vi "insert_doubles_array_example.vi"() -> ()   [LabVIEW 2020, in "Data.PG.lvclass"]
uses:
  Data.PG.lvclass
panel:
  in  "How many points":i32
  in  "Data.PG in":refnum<class "Data.PG.lvclass">
  out "Data.PG out":refnum<class "Data.PG.lvclass">
  in  "milliseconds to wait between points":u32
  in  "paths":string[](array[string])
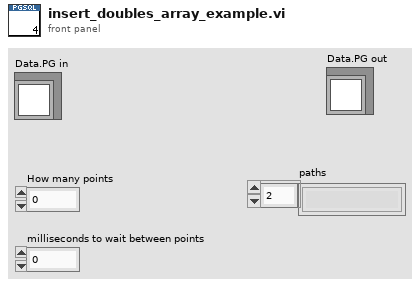
[diagram p1: front panel]
types:
  T1 = cluster{"host":string, "port":string, "user":string, "dbname":string, "password":string}
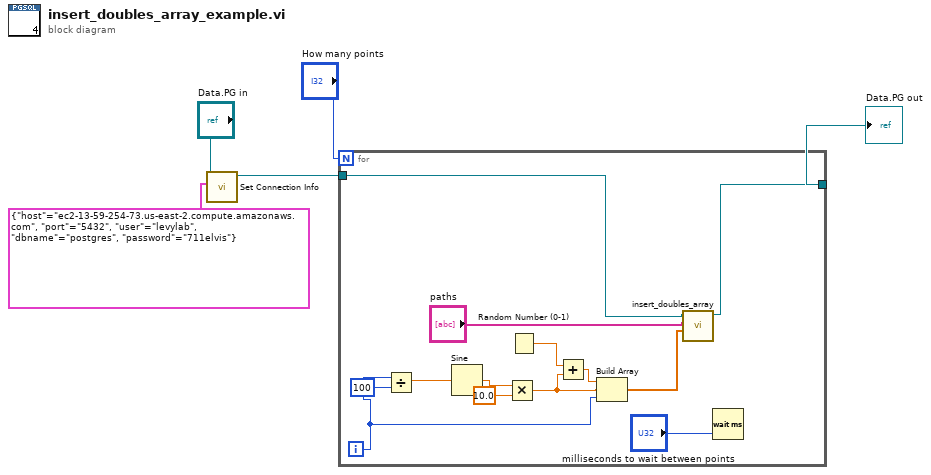
[diagram p0: block diagram]
diagram:
  n1 = call "Set Connection Info.vi"("connection info"=T1 {"host"="ec2-13-59-254-73.us-east-2.compute.amazonaws.com", "port"="5432", "user"="levylab", "dbname"="postgres", "password"="711elvis"}, "Data.PG in"="Data.PG in") -> ("Data.PG out"=w3:refnum<class "Data.PG.lvclass">)  [unwired: 8 in, 1 out]
  n2 = for {
    N: "How many points" -> [_]
    tunnel: w3 -> [w9]
    tunnel: [w6] -> w2
    i -> [w10]
    n3 = Divide(x=w10, y=100) -> (x/y=w18:dbl)
    n4 = Sine(x=w18) -> (sin(x)=w16:dbl)
    n5 = Multiply(x=w16, y=10.0) -> (x*y=w11:dbl)
    n6 = Random Number (0-1)() -> (number: 0 to 1=w14:dbl)
    n7 = Add(x=w14, y=w11) -> (x+y=w12:dbl)
    n8 = Build Array(w12, w11, w10) -> (w7:dbl[])
    n9 = call "insert_doubles_array.vi"("Values"=w7, "paths"="paths", "Data.PG in"=w9) -> ("Data.PG out"=w6:refnum<class "Data.PG.lvclass">)  [unwired: 7 in, 1 out]
    n10 = Wait (ms)(milliseconds to wait="milliseconds to wait between points") -> ()  [unwired: 1 out]
  }
  "Data.PG out" <- w2
